vi "RLT Setup Pannel.vi"() -> (8 "RLT Setup Out":T1={"Degree Setting(F)"=58.0, "Com Setting"=TRUE, "EEV Limit"=500.0, "Thermal Limit"=260.0, "Num Draws (A)"=0, "Draw Amount (GAL)"=15.0, "Num Draws (B)"=0, "Num Draws (C)"=0, "Num Draws (D)"=0})   [LabVIEW 2011]
panel:
  in  "stop":bool
  in  "RLT Setup":T1={"Degree Setting(F)"=58.0, "Com Setting"=TRUE, "EEV Limit"=500.0, "Thermal Limit"=260.0, "Num Draws (A)"=0, "Draw Amount (GAL)"=15.0, "Num Draws (B)"=0, "Num Draws (C)"=0, "Num Draws (D)"=0}
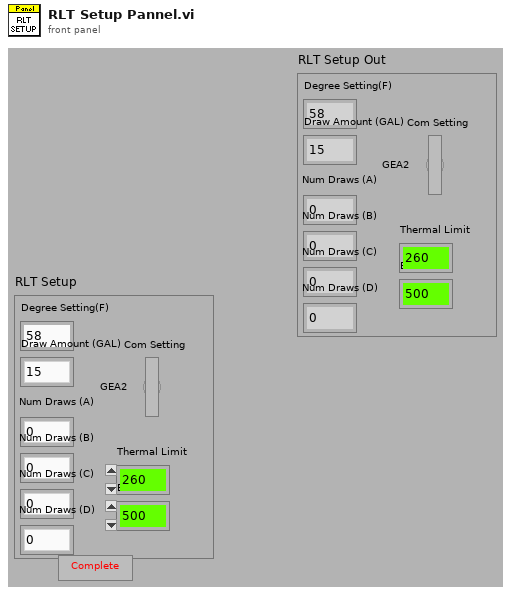
[diagram p1: front panel]
types:
  T1 = cluster{"Degree Setting(F)":dbl, "Com Setting":bool, "EEV Limit":dbl, "Thermal Limit":dbl, "Num Draws (A)":i32, "Draw Amount (GAL)":dbl, "Num Draws (B)":i32, "Num Draws (C)":i32, "Num Draws (D)":i32}
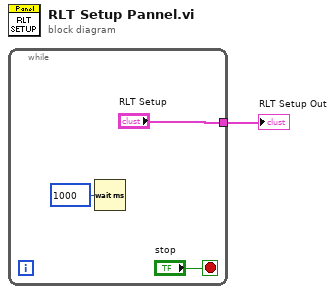
[diagram p0: block diagram]
diagram:
  n1 = while {
    tunnel: ["RLT Setup"] -> w1
    stop <- "stop" stop-if-true
    n2 = Wait (ms)(milliseconds to wait=u32 1000) -> ()  [unwired: 1 out]
  }
  "RLT Setup Out" <- w1
